vi "Project.vi"() -> ()   [LabVIEW 2019]
panel:
  in  "Threshold":dbl
  in  "Tap Inflow":dbl(slide) scale=0.0..10.0
  out "Motor ON":bool
  in  "Tap Flowrate":dbl(slide) scale=0.0..10.0
  out "Tank":dbl(slide) scale=0.0..10.0
  in  "stop":bool
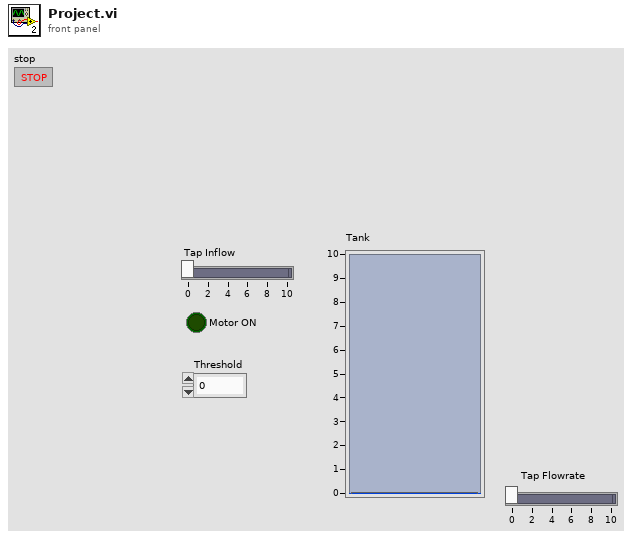
[diagram p1: front panel]
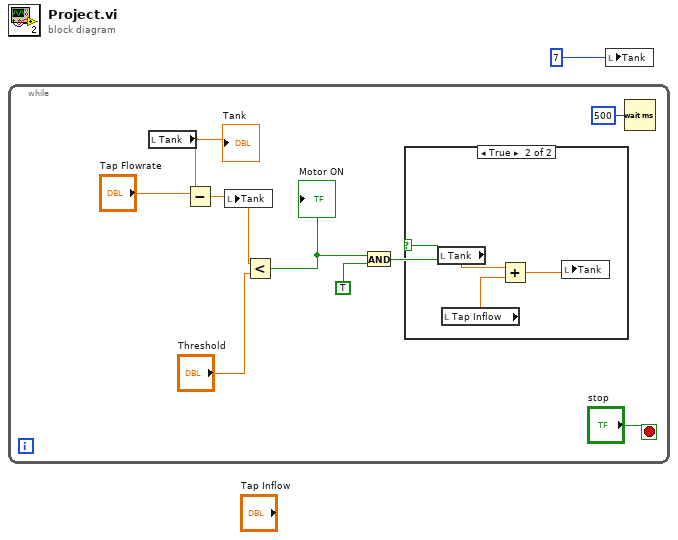
[diagram p0: block diagram]
diagram:
  n1 = while {
    stop <- "stop" stop-if-true
    n2 = local read "Tank"() -> (w7:dbl)
    "Tank" <- w7
    n3 = Subtract(x=w7, y="Tap Flowrate") -> (x-y=w6:dbl)
    n4 = local write "Tank"(w6) -> ()
    n5 = Less?(x=w6, y="Threshold") -> (x < y?=w5:bool)
    "Motor ON" <- w5
    n6 = And(x=w5, y=TRUE) -> (x .and. y?=w3:bool)
    n7 = case shown="True" w3 {
      frame False {
      }
      frame True {
        n8 = local read "Tank"() -> (w13:dbl)
        n9 = local read "Tap Inflow"() -> (w11:dbl)
        n10 = Add(x=w13, y=w11) -> (x+y=w12:dbl)
        n11 = local write "Tank"(w12) -> ()
      }
    }
    n12 = Wait (ms)(milliseconds to wait=u32 500) -> ()  [unwired: 1 out]
  }
  n13 = local write "Tank"(7) -> ()
